vi "Set Title.vi"(8 "error in (no error)":errorcluster, 10 "GUI ref in":refnum<vi>, 11 "Common GUI v3 in":refnum<class "Common GUI v3.lvclass">) -> (0 "error out":errorcluster, 2 "GUI ref out":refnum<vi>, 3 "Common GUI v3 out":refnum<class "Common GUI v3.lvclass">)   [LabVIEW 2026, in "TALOS.lvlib" / "Common GUI v3.lvlib" / "Common GUI v3.lvclass"]
uses:
  Common GUI v3.lvclass
  <vilib>/Utility/error.llb/Trim Whitespace (string).vi
  <vilib>/Utility/error.llb/Trim Whitespace One-Sided.vi
  Support VIs/Global Memory.vi
  TALOS.lvlib
  <vilib>/Utility/LVLibp/NI_PackedLibraryUtility.lvlib
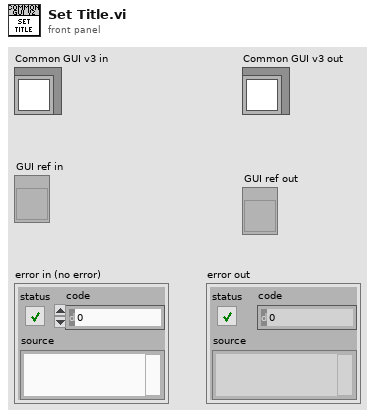
[diagram p1: front panel]
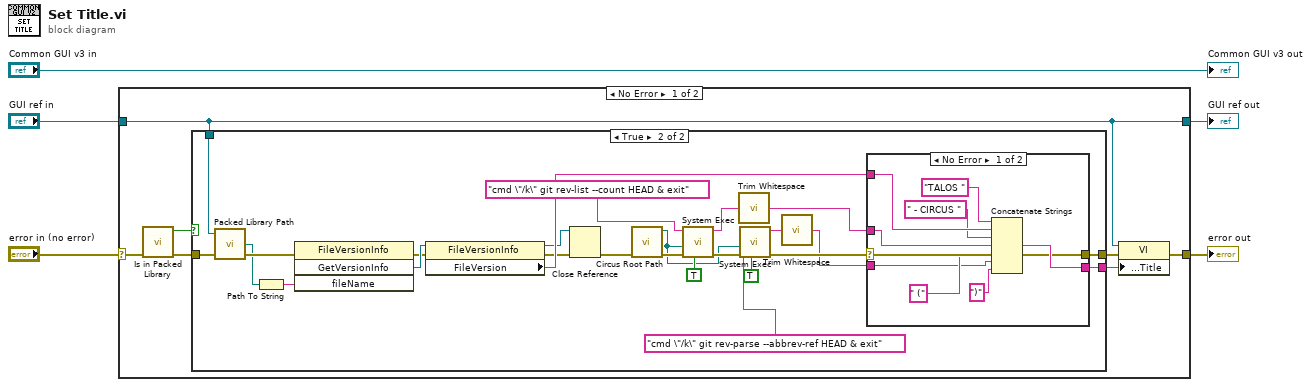
[diagram p0: block diagram]
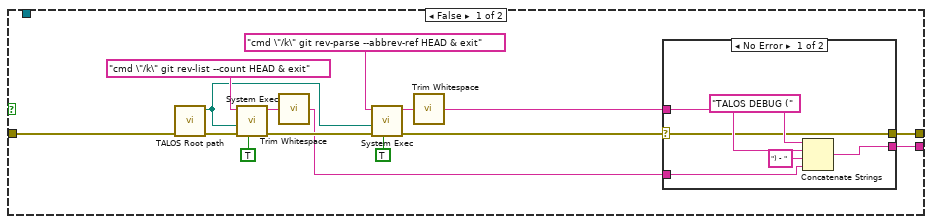
[diagram p2: hidden frame]
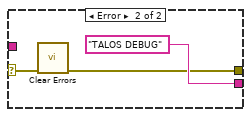
[diagram p3: hidden frame]
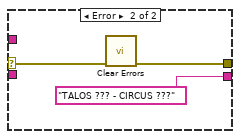
[diagram p4: hidden frame]
diagram:
  n1 = case shown="No Error" "error in (no error)" {
    selector: "error in (no error)" -> [w11 w75]
    tunnel: [w12 w75] -> w5
    tunnel: "GUI ref in" -> [w6 w74]
    tunnel: [w6 w74] -> w1
    frame No Error {
      n2 = call "Is in Packed Library.vi"("error in (no error)"=w11) -> ("error out"=w9:errorcluster, "Is In Packed Library"=w10:bool)  [unwired: 9 in]
      n3 = case shown="True" w10 {
        tunnel: w9 -> [w23 w61]
        tunnel: w6 -> [_ w60]
        tunnel: [w27 w53] -> w8
        tunnel: [w21 w52] -> w7
        frame False {
          n4 = call "TALOS Root path.vi"("error in (no error)"=w23) -> ("error out"=w22:errorcluster, "TALOS Root Path"=w16:path)  [unwired: 9 in]
          n5 = call <vilib>:"System Exec.vi"("run minimized? (F)"=TRUE, "error in (no error)"=w22, "working directory"=w16, "command line"="cmd \"/k\" git rev-list --count HEAD & exit") -> ("error out"=w17:errorcluster, "standard output"=w26:string)  [unwired: 4 in, 2 out]
          n6 = call-poly <vilib>:"Trim Whitespace.vi"("string"=w26) -> ("trimmed string"=w14:string)  [unwired: 1 in]
          n7 = call <vilib>:"System Exec.vi"("run minimized? (F)"=TRUE, "error in (no error)"=w17, "working directory"=w16, "command line"="cmd \"/k\" git rev-parse --abbrev-ref HEAD & exit") -> ("error out"=w13:errorcluster, "standard output"=w18:string)  [unwired: 4 in, 2 out]
          n8 = call-poly <vilib>:"Trim Whitespace.vi"("string"=w18) -> ("trimmed string"=w15:string)  [unwired: 1 in]
          n9 = case shown="No Error" w13 {
            selector: w13 -> [w31 w35]
            tunnel: [w30 "TALOS DEBUG"] -> w27
            tunnel: [w31 w34] -> w21
            tunnel: w15 -> [w32 _]
            tunnel: w14 -> [w28 _]
            frame No Error {
              n10 = Concatenate Strings("TALOS DEBUG (" ("string"), w32, ") - " ("string"), w28) -> (w30:string)
            }
            frame Error {
              n11 = call <vilib>:"Clear Errors.vi"("error in (no error)"=w35) -> ("error out"=w34:errorcluster)  [unwired: 5 in, 1 out]
            }
          }
        }
        frame True {
          n12 = call <vilib>:"Packed Library Path.vi"("error in (no error)"=w61, "vi reference"=w60) -> ("error out"=w56:errorcluster, "packed library path"=w55:path)  [unwired: 1 in, 1 out]
          n13 = Path To String(path=w55) -> (string=w57:string)
          n14 = invoke class="FileVersionInfo" method="GetVersionInfo"(error in=w56, "fileName"=w57) -> (error out=w58:errorcluster, "GetVersionInfo"=w59:refnum<k24>)  [unwired: 2 in, 2 out]
          n15 = property class="FileVersionInfo"(reference=w59, error in=w58) -> (reference out=w45:refnum<k24>, error out=w44:errorcluster, "FileVersion"=w54:string)
          n16 = Close Reference(reference=w45, error in (no error)=w44) -> (error out=w47:errorcluster)
          n17 = call "Circus Root Path.vi"("error in (no error)"=w47) -> ("error out"=w50:errorcluster, "Circus Root Path"=w39:path)  [unwired: 9 in]
          n18 = call <vilib>:"System Exec.vi"("run minimized? (F)"=TRUE, "error in (no error)"=w50, "working directory"=w39, "command line"="cmd \"/k\" git rev-list --count HEAD & exit") -> ("error out"=w40:errorcluster, "standard output"=w51:string)  [unwired: 4 in, 2 out]
          n19 = call-poly <vilib>:"Trim Whitespace.vi"("string"=w51) -> ("trimmed string"=w46:string)  [unwired: 1 in]
          n20 = call <vilib>:"System Exec.vi"("run minimized? (F)"=TRUE, "error in (no error)"=w40, "working directory"=w39, "command line"="cmd \"/k\" git rev-parse --abbrev-ref HEAD & exit") -> ("error out"=w38:errorcluster, "standard output"=w43:string)  [unwired: 4 in, 2 out]
          n21 = call-poly <vilib>:"Trim Whitespace.vi"("string"=w43) -> ("trimmed string"=w37:string)  [unwired: 1 in]
          n22 = case shown="No Error" w38 {
            selector: w38 -> [w66 w72]
            tunnel: w54 -> [w69 _]
            tunnel: [w67 "TALOS ??? - CIRCUS ???"] -> w53
            tunnel: [w66 w71] -> w52
            tunnel: w46 -> [w65 _]
            tunnel: w37 -> [w63 _]
            frame No Error {
              n23 = Concatenate Strings("TALOS " ("string"), w69, " - CIRCUS " ("string"), w65, " (" ("string"), w63, ")" ("string")) -> (w67:string)
            }
            frame Error {
              n24 = call <vilib>:"Clear Errors.vi"("error in (no error)"=w72) -> ("error out"=w71:errorcluster)  [unwired: 5 in, 1 out]
            }
          }
        }
      }
      n25 = property class="VI"(reference=w6, error in=w7, "Front Panel.Title"=w8) -> (error out=w12:errorcluster)  [unwired: 1 out]
    }
    frame Error {
    }
  }
  "error out" <- w5
  "GUI ref out" <- w1
  "Common GUI v3 out" <- "Common GUI v3 in"
